vi "K_30c Wait.vi"(8 "error in (no error)":errorcluster caption="Fehler (Eingang - kein Fehler)", 9 "Zu wartende ms":u32) -> (0 "error out":errorcluster caption="Fehler (Ausgang)")   [LabVIEW 2012]
panel:
  # "Simple wait\nV1.0, b.v."
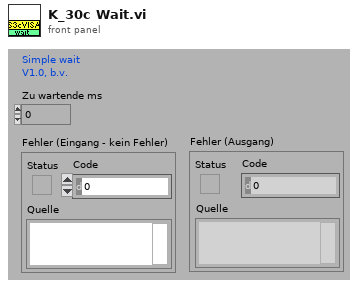
[diagram p1: front panel]
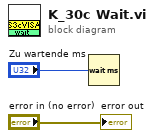
[diagram p0: block diagram]
diagram:
  n1 = Wait (ms)(milliseconds to wait="Zu wartende ms") -> ()  [unwired: 1 out]
  "error out" <- "error in (no error)"
